vi "CheckAllPorts.vi"(11 "Ports":refnum<vi>) -> (3 "Ports":string[][](array[string]))   [LabVIEW 2016]
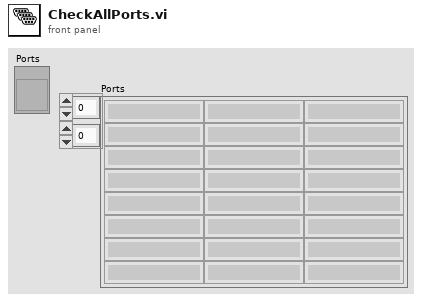
[diagram p1: front panel]
types:
  T1 = cluster{"Port Name":string, "Your Name":string}[]
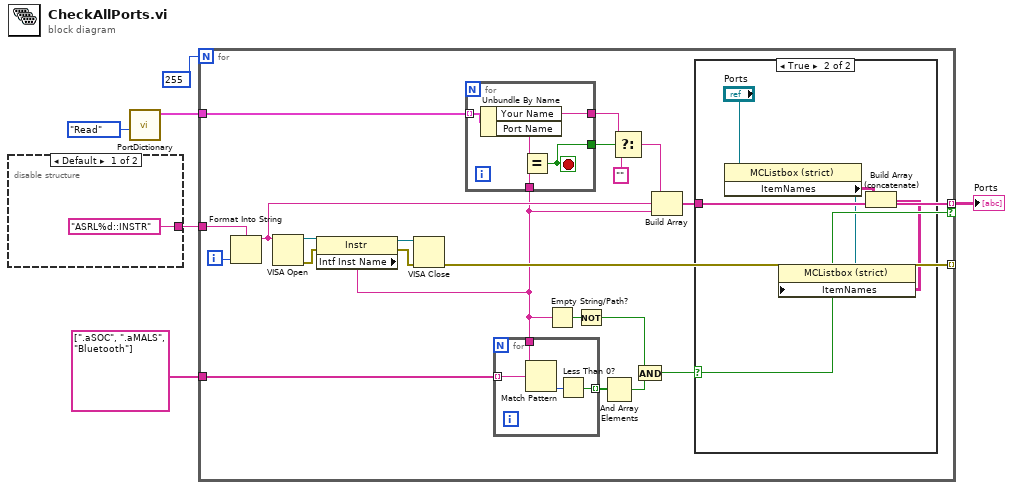
[diagram p0: block diagram]
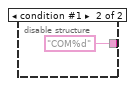
[diagram p2: hidden frame]
diagram:
  n1 = disable-structure shown="Default" {
    disable-tunnel: ["ASRL%d::INSTR" ("format string") "COM%d" ("format string")] -> w5
    frame condition #0 (active) {
    }
    frame condition #1 {
    }
  }
  n2 = call "PortDictionary.vi"("Tasks"=enum16{"Read", "Write"}."Read") -> ("Ports out"=w6:T1)  [unwired: 10 in]
  n3 = for {
    N: 255 -> [_]
    tunnel: [w27] -> _ mode=indexing
    tunnel: string[] [".aSOC", ".aMALS", "Bluetooth"] -> [w25]
    tunnel: w5 -> [w20]
    tunnel: [w10] -> w1 mode=indexing if=w11
    tunnel: w6 -> [w18]
    i -> [w9]
    n4 = Format Into String(format string=w20, w9) -> (resulting string=w19:string)  [unwired: 2 in, 1 out]
    n5 = VISA Open(VISA resource name=w19) -> (VISA resource name=w29:refnum<visa-resource-name>, error out=w12:errorcluster)  [unwired: 4 in]
    n6 = property class="Instr"(reference=w29, error in=w12) -> (reference out=w28:refnum<visa-resource-name>, error out=w26:errorcluster, "Intf Inst Name"=w13:string)
    n7 = VISA Close(VISA resource name=w28, error in (no error)=w26) -> (error out=w27:errorcluster)
    n8 = for {
      tunnel: w18 -> [w39] mode=indexing
      tunnel: [w38] -> w16
      tunnel: w13 -> [w36]
      tunnel: [w35] -> w17
      stop <- w35 stop-if-true
      n9 = Unbundle By Name(w39) -> ("Your Name"=w38:string, "Port Name"=w37:string)
      n10 = Equal?(x=w37, y=w36) -> (x = y?=w35:bool)
    }
    n11 = for {
      tunnel: w13 -> [w43]
      tunnel: w25 -> [w42] mode=indexing
      tunnel: [w40] -> w24 mode=indexing
      n12 = Match Pattern(string=w43, regular expression=w42) -> (offset past match=w41:i32)  [unwired: 1 in, 3 out]
      n13 = Less Than 0?(x=w41) -> (x < 0?=w40:bool)
    }
    n14 = Empty String/Path?(string/path=w13) -> (empty?=w23:bool)
    n15 = Not(x=w23) -> (.not. x?=w21:bool)
    n16 = And Array Elements(Boolean array=w24) -> (logical AND=w22:bool)
    n17 = Select(t=w16, s=w17, f="") -> (s? t:f=w15:string)
    n18 = And(x=w21, y=w22) -> (x .and. y?=w11:bool)
    n19 = Build Array(w15, w19, w13) -> (w10:string[])
    n20 = case shown="True" w11 {
      tunnel: w10 -> [_ w34]
      frame False {
      }
      frame True {
        n21 = property on="Property Node" class="MCListbox (strict)"(reference="Ports") -> (reference out=w32:refnum<vi>, "ItemNames"=w30:string[][])  [unwired: 1 in, 1 out]
        n22 = Build Array (concatenate)(w30, w34) -> (w33:string[][])
        n23 = property on="Property Node" class="MCListbox (strict)"(reference=w32, "ItemNames"=w33) -> ()  [unwired: 1 in, 2 out]
      }
    }
  }
  "Ports" <- w1
